vi "Deserialise content.vi"(8 "error in (no error)":errorcluster, 10 "JSON String to decode":string, 11 "object in":refnum<class "display_data Message.lvclass">) -> (0 "error out":errorcluster, 3 "object out":refnum<class "display_data Message.lvclass">)   [LabVIEW 2018, in "ClientMessaging.lvlib" / "display_data Message.lvclass"]
uses:
  display_data Message.lvclass
  display_data Message.lvclass/display_data Message.ctl
  07040036-bfa6-4fa4-8f98-2b3e398c6dea.vi
  9ae6c6ff-9a0c-48c4-8d84-025a40408b76.vi
  11f3a602-b893-478b-aa2e-4a7e36e09e79.vi
  07040036-bfa6-4fa4-8f98-2b3e398c6dea.vi/e78e2481-545a-4f11-b696-5440e2d36fbe.vi
  07040036-bfa6-4fa4-8f98-2b3e398c6dea.vi/0882be0c-5a6b-41d1-8392-64ed614280b3.vi
  9ae6c6ff-9a0c-48c4-8d84-025a40408b76.vi/737d9989-2182-43ba-9f37-2f2e5bdcf82a.vi
  9ae6c6ff-9a0c-48c4-8d84-025a40408b76.vi/5dac1ee3-f109-4ff8-920e-fb3c383fab37.vi
  11f3a602-b893-478b-aa2e-4a7e36e09e79.vi/dbc59782-526d-440d-ae4d-dcc300f07bd2.vi
  11f3a602-b893-478b-aa2e-4a7e36e09e79.vi/ae71eb5f-5241-43d2-a4f1-93e712d0c2ed.vi
  <userlib>/_OpenG.lib/lvdata/lvdata.llb/Get Cluster Element by Name__ogtk.vi
  <userlib>/_OpenG.lib/lvdata/lvdata.llb/Get Cluster Element Names__ogtk.vi
  Base Classes/Message Class/Message Class.lvclass
  <vilib>/wsapi/NI_WebServices.lvlib
  ClientMessaging.lvlib
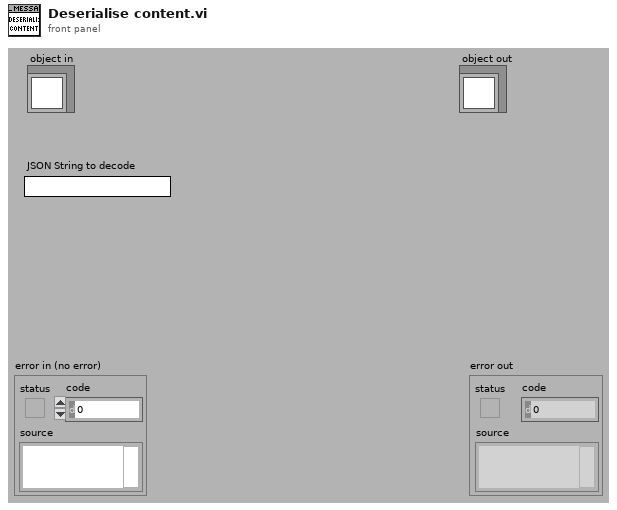
[diagram p1: front panel]
types:
  T1 = typedef "imagedata.ctl" = cluster{"image type":i32, "image depth":i32, "image":u8[], "mask":u8[], "colors":u32[], "Rectangle":cluster{"left":i16, "top":i16, "right":i16, "bottom":i16}}
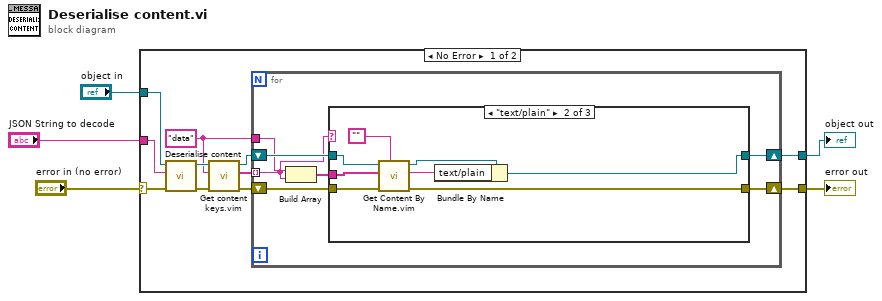
[diagram p0: block diagram]
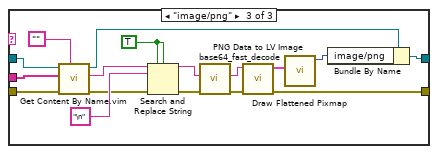
[diagram p3: hidden frame]
diagram:
  n1 = case shown="No Error" "error in (no error)" {
    selector: "error in (no error)" -> [w14 w52]
    tunnel: [w15 w52] -> w4
    tunnel: [w16 w51] -> w2
    tunnel: "object in" -> [w13 w51]
    tunnel: "JSON String to decode" -> [w12 _]
    frame No Error {
      w6 = "data" ("Key Name (default \"\": content keys)")
      n2 = call-parent "Deserialise content.vi"("error in (no error)"=w14, "JSON String to decode"=w12, "object in"=w13) -> ("error out"=w10:errorcluster, "object out"=w11:refnum<class "display_data Message.lvclass">)  [unwired: 7 in]
      n3 = call "Get content keys.vim"("error in (no error)"=w10, "Key Name (default \"\": content keys)"=w6, "object in"=w11) -> ("error out"=w7:errorcluster, "Key names"=w8:string[], "object out"=w9:refnum<class "display_data Message.lvclass">)  [unwired: 6 in]
      n4 = for {
        shift-right: [w22] -> w15
        shift-left: w7 -> [w23]
        tunnel: w8 -> [w19] mode=indexing
        shift-right: [w21] -> w16
        shift-left: w9 -> [w20]
        tunnel: w6 -> [w18]
        n5 = Build Array(w18, w19) -> (w17:string[])
        n6 = case shown="\"text/plain\"" w19 {
          tunnel: w23 -> [w24 w27 w38]
          tunnel: [w24 w28 w47] -> w22
          tunnel: [w25 w33 w49] -> w21
          tunnel: w20 -> [w25 w32 w40]
          tunnel: w17 -> [_ w26 w34]
          frame "0", Default {
          }
          frame "text/plain" {
            n7 = call "Get Content By Name.vim"("Type of content"="", "error in (no error)"=w27, "Name of Content Item"=w26, "Message In"=w32) -> ("error out"=w28:errorcluster, "Data Out"=w30:string, "Message Out"=w29:refnum<class "display_data Message.lvclass">)  [unwired: 5 in]
            n8 = Bundle By Name(cluster=w29, "text/plain"=w30) -> (w33:refnum<class "display_data Message.lvclass">)
          }
          frame "image/png" {
            w42 = TRUE ("ignore case? (F)")
            n9 = call "Get Content By Name.vim"("Type of content"="", "error in (no error)"=w38, "Name of Content Item"=w34, "Message In"=w40) -> ("error out"=w37:errorcluster, "Data Out"=w36:string, "Message Out"=w39:refnum<class "display_data Message.lvclass">)  [unwired: 5 in]
            n10 = Search and Replace String(replace all?=w42, case sensitive?=w42, input string=w36, search string="\n", error in=w37) -> (result string=w44:string, error out=w41:errorcluster)  [unwired: 3 in, 2 out]
            n11 = call "base64_fast_decode.vi"("error in (no error)"=w41, "string in (base64-encoded)"=w44) -> ("error out"=w45:errorcluster, "string out (decoded)"=w46:string)  [unwired: 8 in]
            n12 = call <vilib>:"PNG Data to LV Image.vi"("error in (no error)"=w45, "png data"=w46) -> ("error out"=w47:errorcluster, "image data"=w50:T1)  [unwired: 8 in]
            n13 = call <vilib>:"Draw Flattened Pixmap.vi"("image data"=w50) -> ("new picture"=w48:picture)  [unwired: 8 in]
            n14 = Bundle By Name(cluster=w39, "image/png"=w48) -> (w49:refnum<class "display_data Message.lvclass">)
          }
        }
      }
    }
    frame Error {
    }
  }
  "error out" <- w4
  "object out" <- w2
